vi "Process Data Conifg PID Gain Save_vel.vi"(5 "에러 입력(에러 없음)":errorcluster, 7 "Pos PID gain 1":T1, 9 "Velocity limit 1":cluster{"output high":dbl, "output low":dbl}, 10 "Pos PID gain 0":T1, 12 "Velocity limit 0":cluster{"output high":dbl, "output low":dbl}) -> (19 "에러 출력":errorcluster)   [LabVIEW 2019]
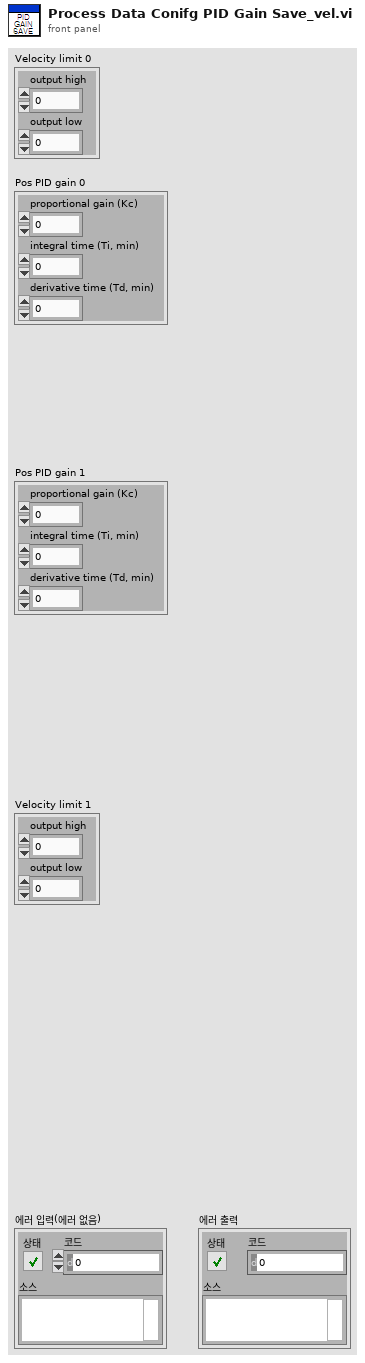
[diagram p1: front panel]
types:
  T1 = cluster{"proportional gain (Kc)":dbl, "integral time (Ti, min)":dbl, "derivative time (Td, min)":dbl}
  T2 = enum16{"open", "replace", "create", "open or create", "replace or create", "replace or create with confirmation"}
  T3 = cluster{"output high":dbl, "output low":dbl, "proportional gain (Kc)":dbl, "integral time (Ti, min)":dbl, "derivative time (Td, min)":dbl, "output high":dbl, "output low":dbl, "proportional gain (Kc)":dbl, "integral time (Ti, min)":dbl, "derivative time (Td, min)":dbl}
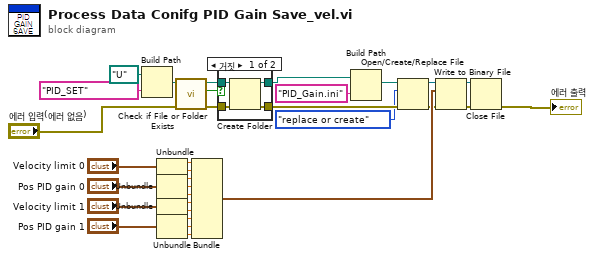
[diagram p0: block diagram]
diagram:
  n1 = Build Path(base path=path "U:/" ("베이스 경로"), name or relative path="PID_SET" ("시간 포맷 문자열 (%c)")) -> (appended path=w1:path)
  n2 = Unbundle("Velocity limit 0") -> ("output high"=w20:dbl, "output low"=w21:dbl)
  n3 = Unbundle("Pos PID gain 0") -> ("proportional gain (Kc)"=w23:dbl, "integral time (Ti, min)"=w24:dbl, "derivative time (Td, min)"=w25:dbl)
  n4 = Unbundle("Velocity limit 1") -> ("output high"=w27:dbl, "output low"=w28:dbl)
  n5 = Unbundle("Pos PID gain 1") -> ("proportional gain (Kc)"=w30:dbl, "integral time (Ti, min)"=w31:dbl, "derivative time (Td, min)"=w32:dbl)
  n6 = call <vilib>:"Check if File or Folder Exists.vi"("error in (no error)"="에러 입력(에러 없음)", "path"=w1) -> ("error out"=w6:errorcluster, "file or folder exists?"=w2:bool, "dup path"=w3:path)  [unwired: 7 in]
  n7 = Bundle("output high"=w20, "output low"=w21, "proportional gain (Kc)"=w23, "integral time (Ti, min)"=w24, "derivative time (Td, min)"=w25, "output high"=w27, "output low"=w28, "proportional gain (Kc)"=w30, "integral time (Ti, min)"=w31, "derivative time (Td, min)"=w32) -> (w17:T3)  [unwired: 1 in]
  n8 = case shown="거짓" w2 {
    tunnel: w3 -> [w36 w38]
    tunnel: [w35 w38] -> w8
    tunnel: w6 -> [w34 w37]
    tunnel: [w33 w37] -> w12
    frame False {
      n9 = Create Folder(path (use dialog)=w36, error in=w34) -> (created path=w35:path, error out=w33:errorcluster)  [unwired: 1 in, 1 out]
    }
    frame True {
    }
  }
  n10 = Build Path(base path=w8, name or relative path="PID_Gain.ini" ("이름 또는 상대 경로")) -> (appended path=w10:path)
  n11 = Open/Create/Replace File(file path (use dialog)=w10, error in=w12, operation (0:open)=T2."replace or create" ("동작(0:open)")) -> (refnum out=w14:refnum<file>, error out=w13:errorcluster)  [unwired: 3 in, 1 out]
  n12 = Write to Binary File(file (use dialog)=w14, data=w17, error in=w13) -> (refnum out=w16:refnum<file>, error out=w15:errorcluster)  [unwired: 3 in, 1 out]
  n13 = Close File(refnum=w16, error in=w15) -> (error out=→"에러 출력":errorcluster)  [unwired: 1 out]
